vi "Keypad.vi"(11 "KeyPad":T1) -> (15 "Keypad Out":dbl)   [LabVIEW 2012]
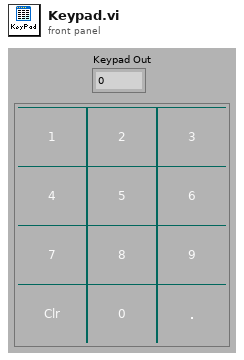
[diagram p1: front panel]
types:
  T1 = cluster{"2":bool, "1":bool, "3":bool, "4":bool, "9":bool, "5":bool, "6":bool, "7":bool, "8":bool, "0":bool, "dp":bool, "Clear":bool}
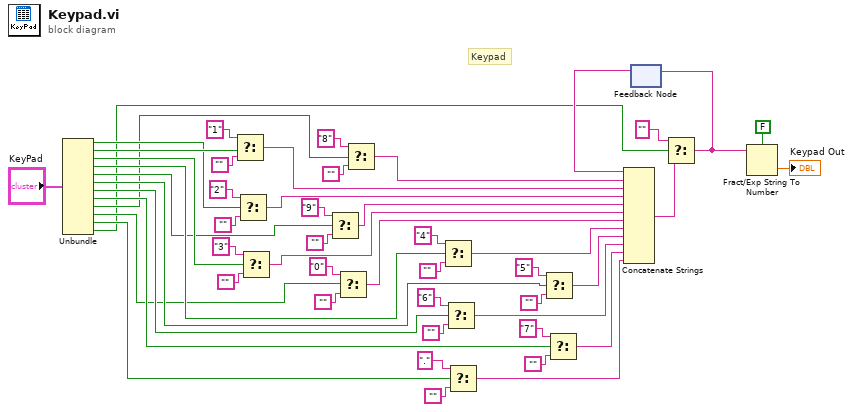
[diagram p0: block diagram]
diagram:
  # "Keypad"
  n1 = Unbundle("KeyPad") -> ("2"=w15:bool, "1"=w16:bool, "3"=w14:bool, "4"=w13:bool, "9"=w12:bool, "5"=w11:bool, "6"=w10:bool, "7"=w9:bool, "8"=w8:bool, "0"=w7:bool, "dp"=w6:bool, "Clear"=w1:bool)
  n2 = Select(t="1", s=w16, f="") -> (s? t:f=w27:string)
  n3 = Select(t="2", s=w15, f="") -> (s? t:f=w26:string)
  n4 = Select(t="3", s=w14, f="") -> (s? t:f=w24:string)
  n5 = Select(t="9", s=w12, f="") -> (s? t:f=w25:string)
  n6 = Select(t="0", s=w7, f="") -> (s? t:f=w23:string)
  n7 = Select(t="8", s=w8, f="") -> (s? t:f=w28:string)
  n8 = Select(t="4", s=w13, f="") -> (s? t:f=w22:string)
  n9 = Select(t="6", s=w10, f="") -> (s? t:f=w20:string)
  n10 = Select(t=".", s=w6, f="") -> (s? t:f=w18:string)
  n11 = Select(t="5", s=w11, f="") -> (s? t:f=w21:string)
  n12 = Select(t="7", s=w9, f="") -> (s? t:f=w19:string)
  n13 = feedback #1() -> (w5:string)  [unwired: 1 in]
  n14 = Concatenate Strings(w5, w28, w27, w26, w25, w24, w23, w22, w21, w20, w19, w18) -> (w30:string)
  n15 = Select(t="", s=w1, f=w30) -> (s? t:f=w4:string)
  n16 = feedback-in #1(w4) -> ()
  n17 = Fract/Exp String To Number(use system decimal point (T)=FALSE, string=w4) -> (number=→"Keypad Out":dbl)  [unwired: 2 in, 1 out]
